vi "Set Current CCD.vi"(8 "error in (no error)":errorcluster, 11 "CCDCamera.lvclass":refnum<class "CCDCamera.lvclass">) -> (0 "error out":errorcluster, 3 "CCDCamera.lvclass 2":refnum<class "CCDCamera.lvclass">)   [LabVIEW 2018, in "CCDCamera.lvclass"]
doc: "This VI reads the camera index of the class and sets the current CCD."
uses:
  CCDCamera.lvclass
  CCDCamera.lvclass/CCDCamera.ctl
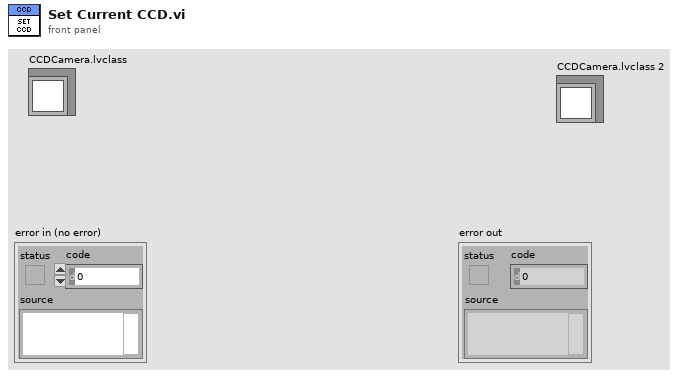
[diagram p1: front panel]
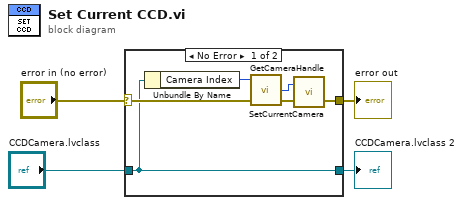
[diagram p0: block diagram]
diagram:
  n1 = case shown="No Error" "error in (no error)" {
    selector: "error in (no error)" -> [w9 w12]
    tunnel: [w8 w12] -> w3
    tunnel: [w6 w11] -> w1
    tunnel: "CCDCamera.lvclass" -> [w6 w11]
    frame No Error {
      n2 = Unbundle By Name(w6) -> ("Camera Index"=w5:u16)
      n3 = call <userlib>:"GetCameraHandle.vi"("error in (no error)"=w9, "cameraIndex"=w5) -> ("error out"=w7:errorcluster, "cameraHandle"=w10:i32)  [unwired: 1 in, 1 out]
      n4 = call <userlib>:"SetCurrentCamera.vi"("error in (no error)"=w7, "cameraHandle"=w10) -> ("error out"=w8:errorcluster)  [unwired: 1 out]
    }
    frame Error {
    }
  }
  "error out" <- w3
  "CCDCamera.lvclass 2" <- w1
